vi "Temperature Controller.vi"() -> ()   [LabVIEW 2019]
uses:
  Units.ctl
  TempController_client/TempController_client Class/RPC Messages/MeasureRequest/MeasureRequest_Data.ctl
  TempController_client/TempController_client Class/RPC Messages/ControllerSettingsRequest/ControllerSettingsRequest_Data.ctl
  TempController_client/TempController_client Class/TempController_client.lvclass
panel:
  in  "Units to display":T1
  in  "Units":T1
  in  "Enable":bool
  in  "Temperature Setpoint":dbl(slide) scale=0.0..200.0
  out "Actuall Temperature":dbl(graph)
  in  "Address":string="localhost:50051"
  # "Temperature Controller Panel"
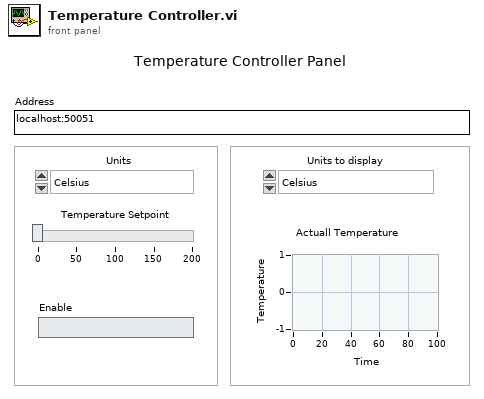
[diagram p1: front panel]
types:
  T1 = typedef "Units.ctl" = enum16{"Celsius", "Fahrenheit"}
  T2 = typedef "TempController_client.lvlib/TempController_client.lvclass/MeasureRequest_Data.ctl" = cluster{"unit":i32}
  T3 = typedef "TempController_client.lvlib/TempController_client.lvclass/ControllerSettingsRequest_Data.ctl" = cluster{"temperature_setpoint":dbl, "unit":i32, "enabled":bool}
  T4 = typedef "TempController_client.lvlib/TempController_client.lvclass/MeasureResponse_Data.ctl" = cluster{"temperature":dbl}
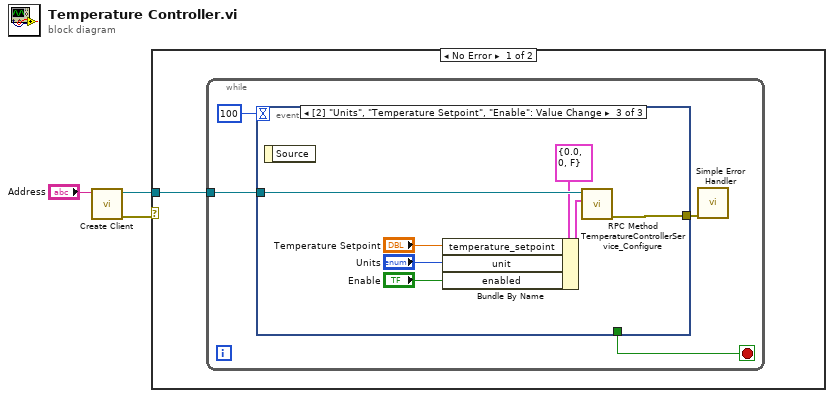
[diagram p0: block diagram]
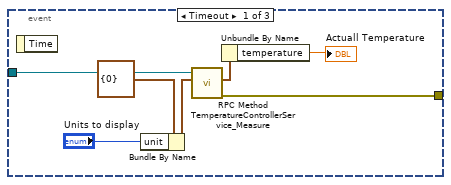
[diagram p2: hidden frame]
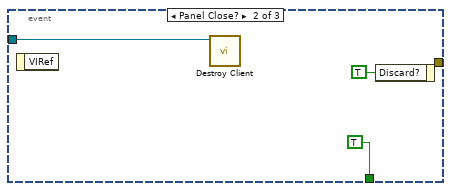
[diagram p3: hidden frame]
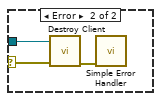
[diagram p4: hidden frame]
diagram:
  n1 = call "Create Client.vi"("address"="Address") -> ("error out"=w1:errorcluster, "gRPC Client out"=w2:refnum<class "TempController_client.lvclass">)  [unwired: 9 in]
  n2 = case shown="No Error" w1 {
    selector: w1 -> [_ w27]
    tunnel: w2 -> [w4 w28]
    frame No Error {
      n3 = while {
        tunnel: w4 -> [w8]
        stop <- w5 stop-if-true
        n4 = event shown="[2] \"Units\", \"Temperature Setpoint\", \"Enable\": Value Change" {
          selector: _ -> [_ _ _]
          dyn-events: _ -> [_ _ _]
          timeout: 100 -> [_ _ _]
          tunnel: w8 -> [w15 w16 w25]
          tunnel: [w11 _ w24] -> w6
          tunnel: [_ TRUE _] -> w5
          event Timeout {
            n5 = event-data() -> ()  [unwired: 1 in, 1 out]
            n6 = Bundle By Name(cluster=T2 {"unit"=0} ("Request Data"), "unit"="Units to display") -> (w13:T2)
            n7 = call "RPC Method TemperatureControllerService_Measure.vi"("Request Data"=w13, "gRPC Client in"=w15) -> ("error out"=w11:errorcluster, "Response Data"=w10:T4)  [unwired: 7 in, 1 out]
            n8 = Unbundle By Name(w10) -> ("temperature"=→"Actuall Temperature":dbl)
          }
          event Panel Close? {
            n9 = event-data() -> ()  [unwired: 1 in, 1 out]
            n10 = call "Destroy Client.vi"("gRPC Client in"=w16) -> ()  [unwired: 9 in, 2 out]
            n11 = event-data("Discard?"=TRUE) -> ()  [unwired: 1 in, 1 out]
          }
          event "Temperature Setpoint", "Enable": Value Change {
            n12 = event-data() -> ()  [unwired: 1 in, 1 out]
            n13 = Bundle By Name(cluster=T3 {"temperature_setpoint"=0.0, "unit"=0, "enabled"=FALSE} ("Request Data"), "temperature_setpoint"="Temperature Setpoint", "unit"="Units", "enabled"="Enable") -> (w22:T3)
            n14 = call "RPC Method TemperatureControllerService_Configure.vi"("Request Data"=w22, "gRPC Client in"=w25) -> ("error out"=w24:errorcluster)  [unwired: 7 in, 2 out]
          }
        }
        n15 = call <vilib>:"Simple Error Handler.vi"("error in (no error)"=w6) -> ()  [unwired: 4 in, 5 out]
      }
    }
    frame Error {
      n16 = call "Destroy Client.vi"("error in (no error)"=w27, "gRPC Client in"=w28) -> ("error out"=w26:errorcluster)  [unwired: 8 in, 1 out]
      n17 = call <vilib>:"Simple Error Handler.vi"("error in (no error)"=w26) -> ()  [unwired: 4 in, 5 out]
    }
  }
